vi "20150818 Main structure.vi"() -> ()   [LabVIEW 2013]
uses:
  <vilib>/Utility/error.llb/Error Cluster From Error Code.vi
  <vilib>/ErrorRing/Error Ring.xnode
  <userlib>/support/Message Queue/Message Queue.lvlib
panel:
  out "Distance(cm)":dbl
  out "UL sensor Initialize OK?":bool
  out "Servo Initialize OK?":bool
  in  "Initialize":bool
  in  "stop":bool
  out "error out":errorcluster
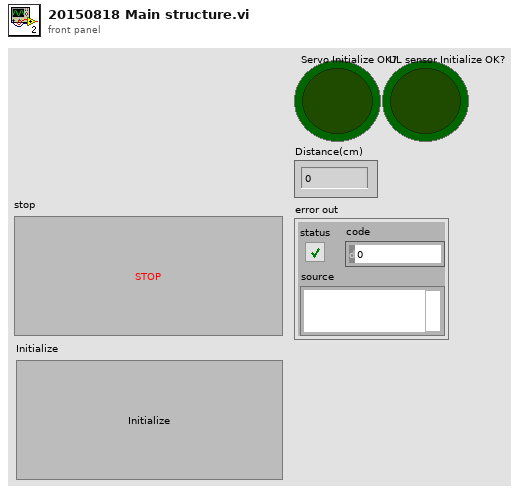
[diagram p1: front panel]
types:
  T1 = typedef "Message Queue.lvlib/All Message Queues.ctl" = cluster{"Actuator":refnum<queue>, "Sensor":refnum<queue>, "Algorithm":refnum<queue>}
  T2 = enum16{"Initialize", "Close", "Set Pulse widths"}
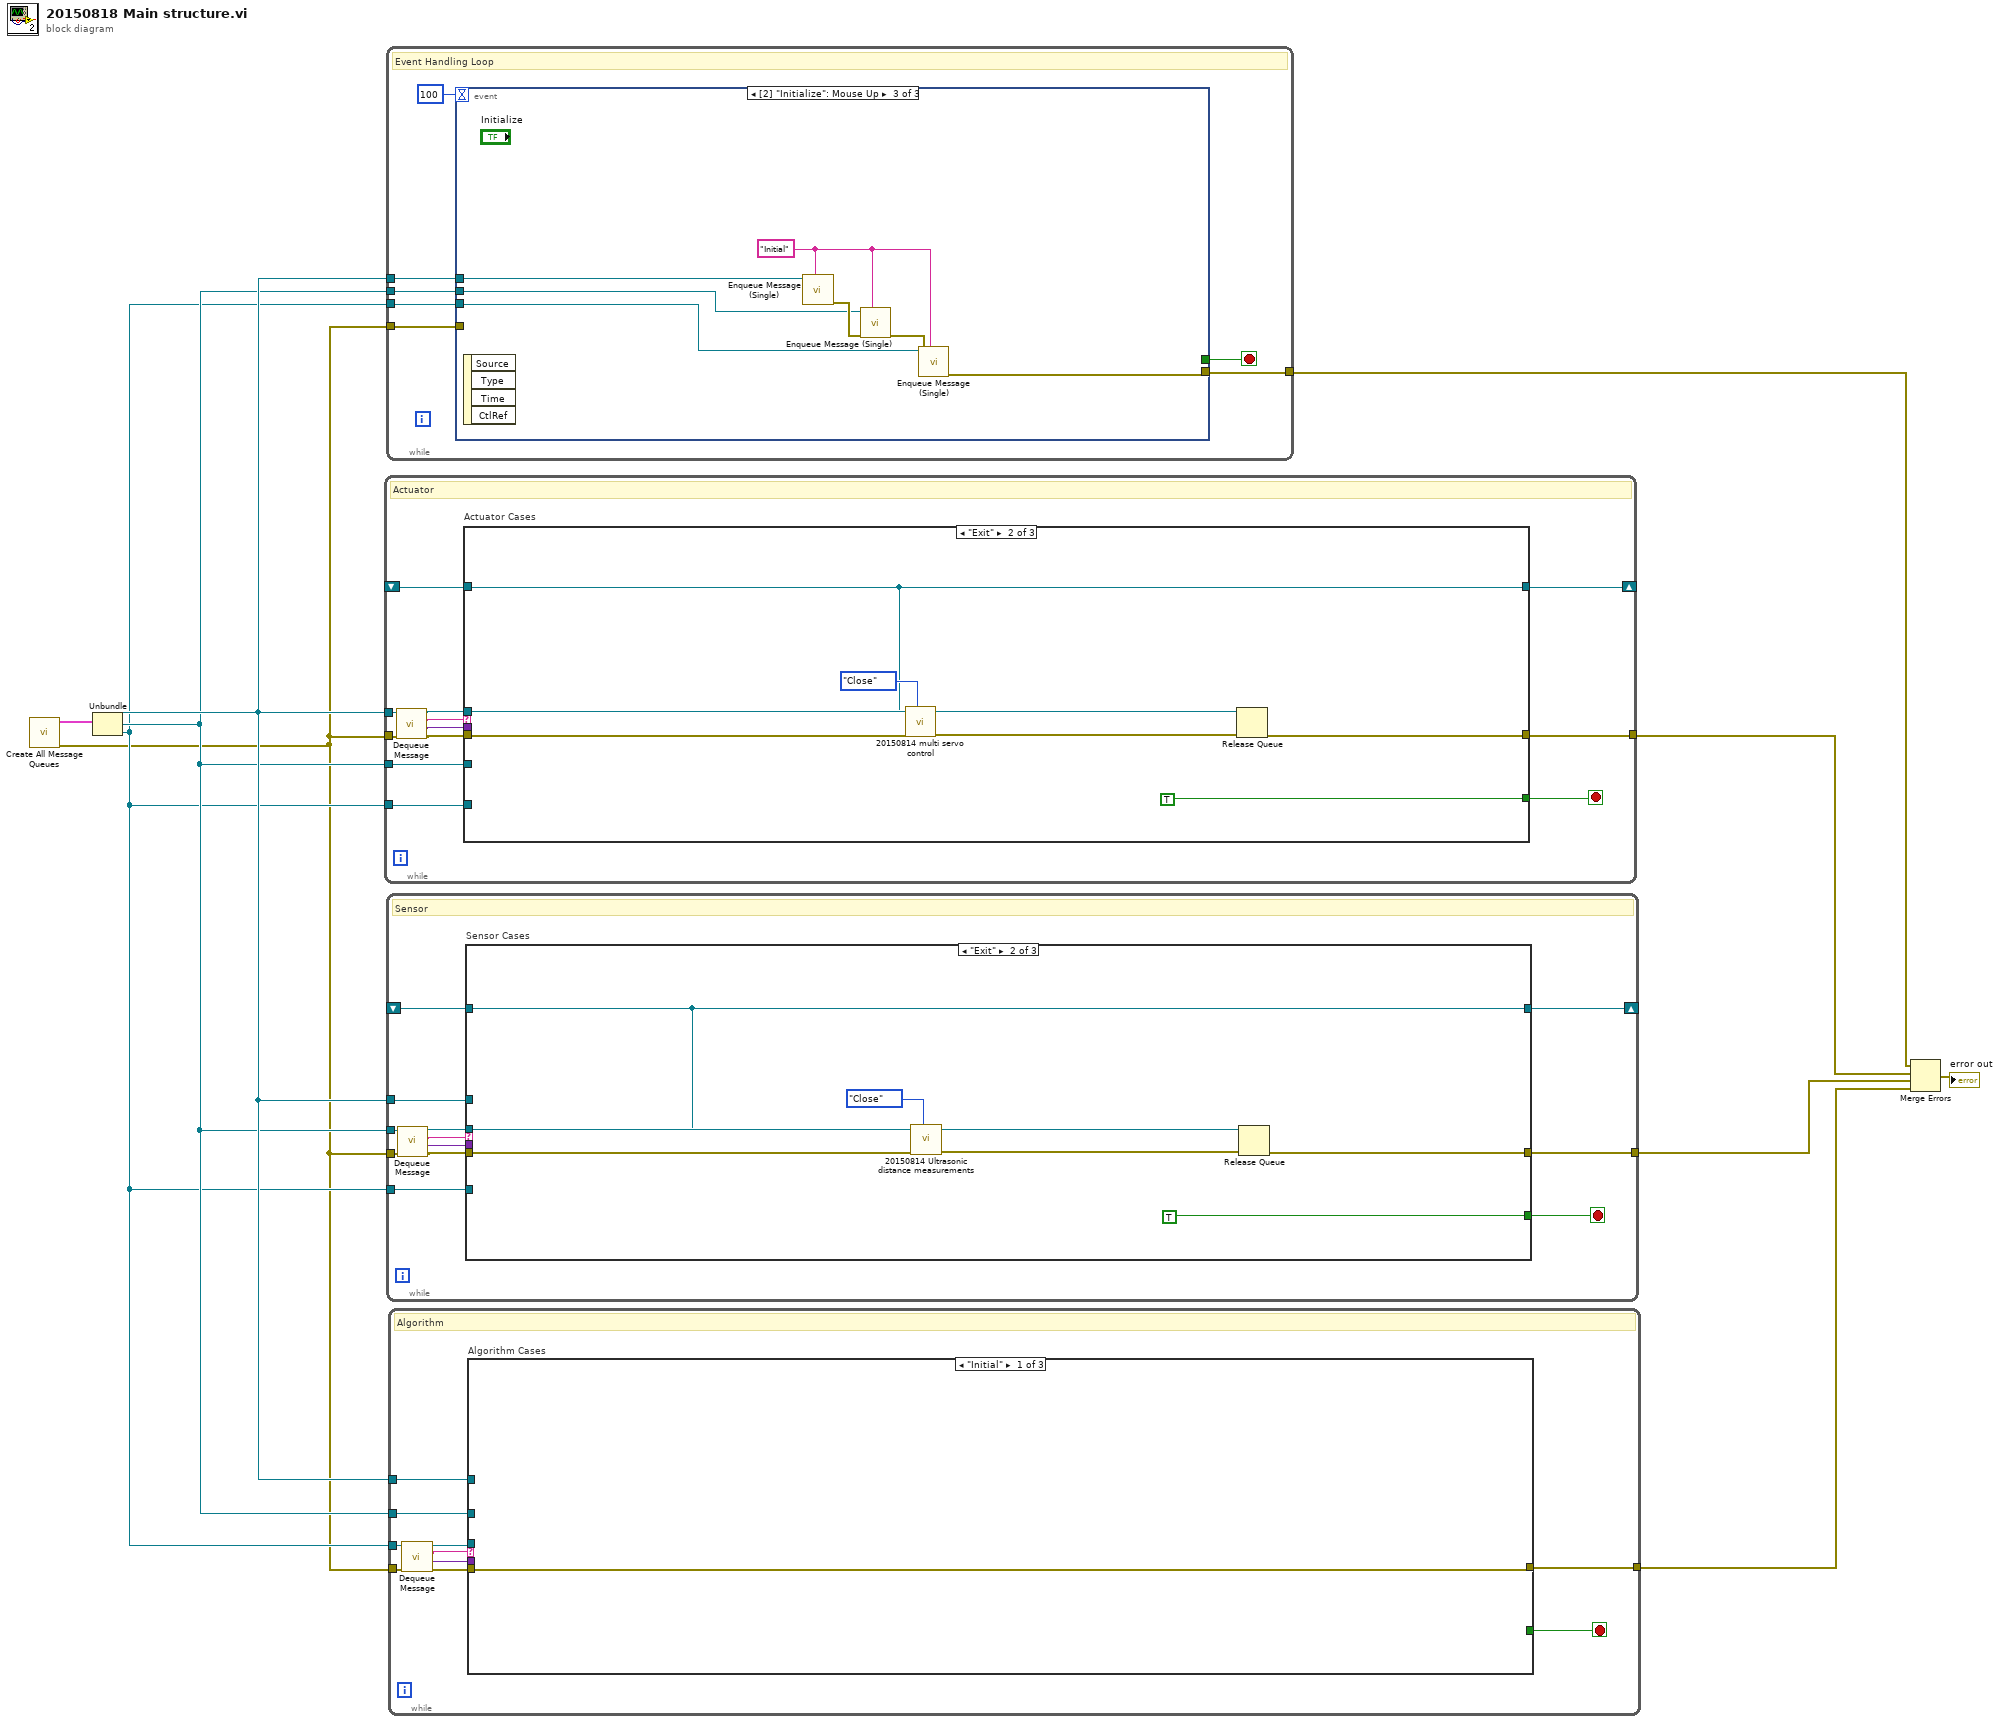
[diagram p0: block diagram]
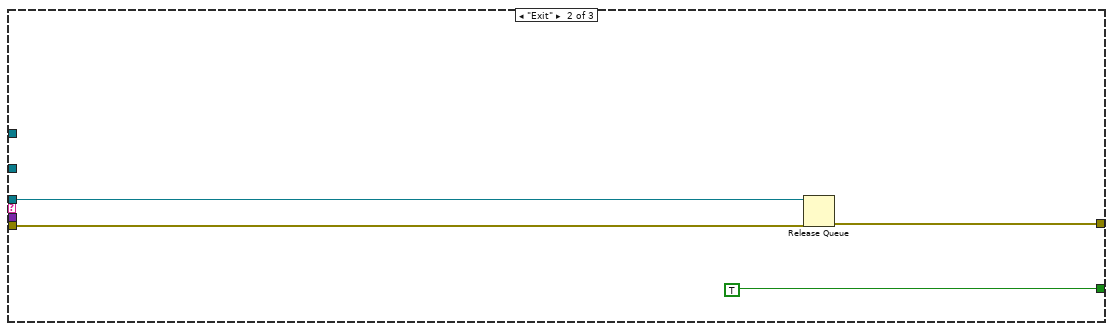
[diagram p2: hidden frame]
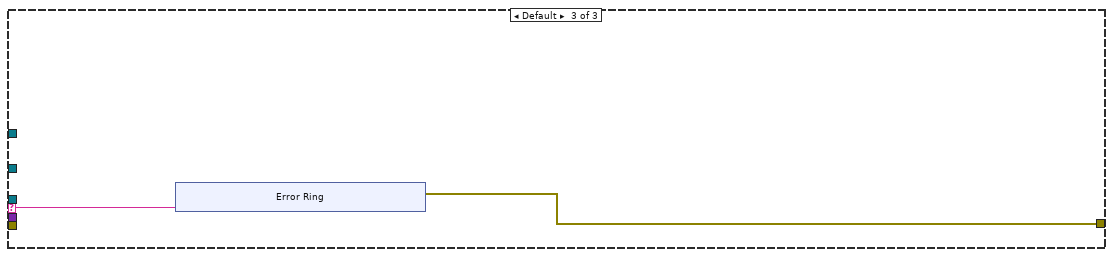
[diagram p3: hidden frame]
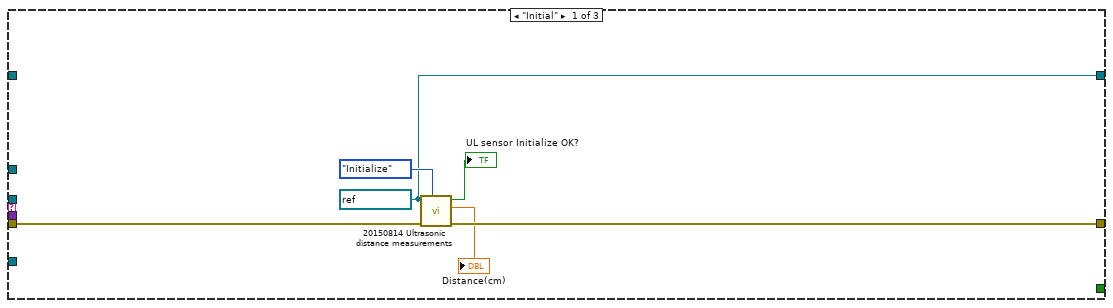
[diagram p4: hidden frame]
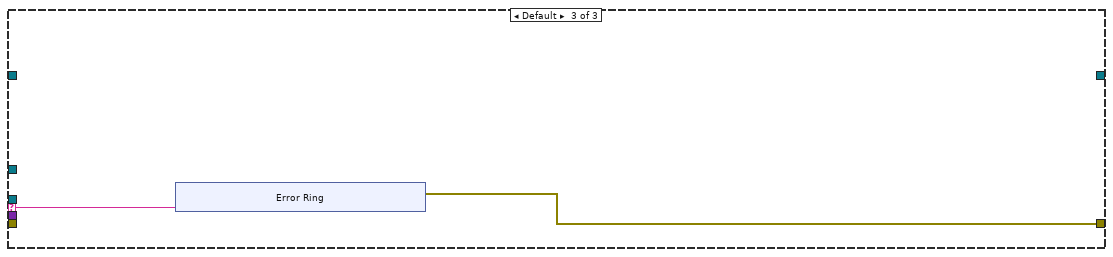
[diagram p5: hidden frame]
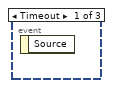
[diagram p6: hidden frame]
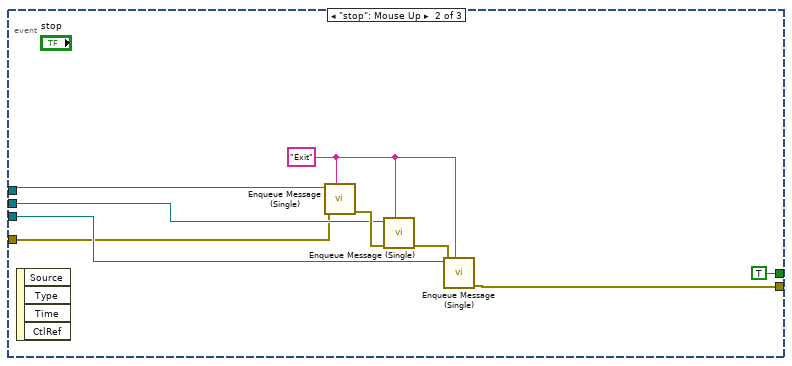
[diagram p7: hidden frame]
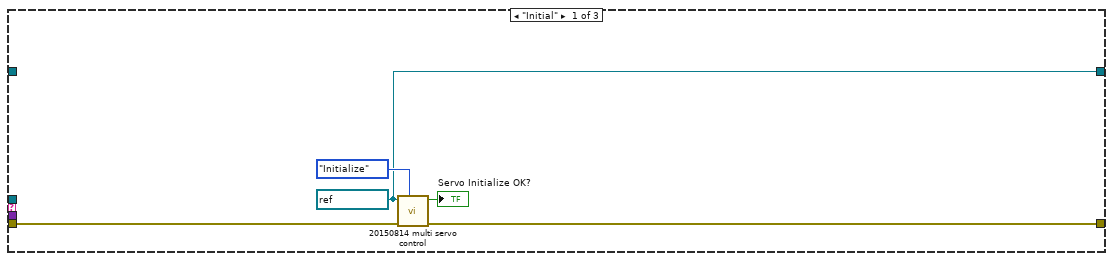
[diagram p8: hidden frame]
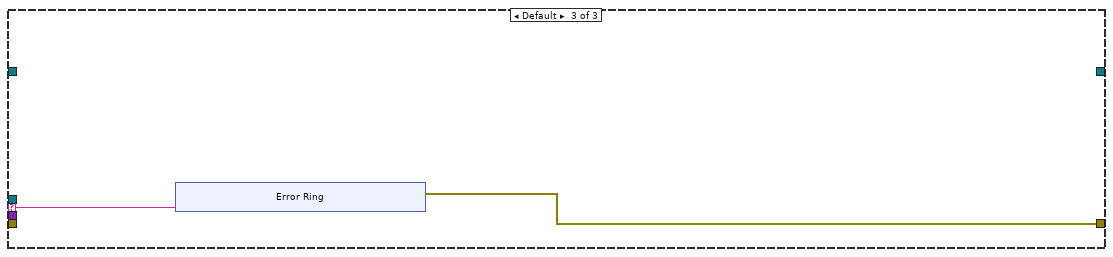
[diagram p9: hidden frame]
diagram:
  n1 = call <userlib>:"Create All Message Queues.vi"() -> ("error out"=w2:errorcluster, "Message Queues out"=w10:T1)  [unwired: 10 in]
  n2 = Unbundle(w10) -> ("Actuator"=w5:refnum<queue>, "Sensor"=w4:refnum<queue>, "Algorithm"=w3:refnum<queue>)
  n3 = while {
    tunnel: [w16] -> w9
    tunnel: w5 -> [w21]
    tunnel: w2 -> [w15]
    tunnel: w4 -> [w14]
    tunnel: w3 -> [w13]
    shift-right: [w12] -> _
    shift-left: _ -> [w11]
    stop <- w22 stop-if-true
    # "Actuator"
    n4 = call <userlib>:"Dequeue Message.vi"("error in (no error)"=w15, "Message Queue"=w21) -> ("error out"=w18:errorcluster, "Message Data"=w19:variant, "Message"=w20:string, "dup Message Queue"=w17:refnum<queue>)  [unwired: 6 in]
    n5 = case "Actuator Cases" shown="\"Exit\"" w20 {
      selector: w20 -> [_ _ w35]
      tunnel: w17 -> [_ w34 _]
      tunnel: w18 -> [w25 w31 _]
      tunnel: [w24 w33 w36] -> w16
      tunnel: [_ TRUE ("Priority Message? (F)") _] -> w22
      tunnel: w19 -> [_ _ _]
      tunnel: w14 -> [_ _ _]
      tunnel: w13 -> [_ _ _]
      tunnel: [w23 w28 _] -> w12
      tunnel: w11 -> [_ w28 _]
      frame "Initial" {
        w23 = refnum<visa-resource-name> "COM10" ("Serial Port")
        # "Initialize - Send separate messages to initialize the data and the front panel.  Bundle control references."
        n6 = call "20150814 multi servo control.vi"("Action"=T2."Initialize", "error in (no error)"=w25, "Serial Port"=w23) -> ("Error Out"=w24:errorcluster, "Initialize OK?"=→"Servo Initialize OK?":bool)  [unwired: 7 in]
      }
      frame "Exit" {
        # "Exit - Exit the application."
        n7 = call "20150814 multi servo control.vi"("Action"=T2."Close", "error in (no error)"=w31, "Serial Port"=w28) -> ("Error Out"=w30:errorcluster)  [unwired: 7 in, 1 out]
        n8 = Release Queue(queue=w34, error in (no error)=w30) -> (error out=w33:errorcluster)  [unwired: 1 in, 2 out]
      }
      frame Default {
        # "'Default' case only runs if there is a message that isn't defined in any of the other cases.  Output a programming error."
        n9 = xnode "Error Ring"("parameter 0"=w35) -> ("error out"=w36:errorcluster)
      }
    }
  }
  n10 = while {
    tunnel: w5 -> [w50]
    tunnel: w4 -> [w46]
    tunnel: w3 -> [w48]
    tunnel: w2 -> [w45]
    tunnel: [w44] -> w1
    stop <- w49 stop-if-true
    # "Event Handling Loop"
    n11 = event shown="[2] \"Initialize\": Mouse Up" {
      selector: _ -> [_ _ _]
      dyn-events: _ -> [_ _ _]
      timeout: 100 -> [_ _ _]
      tunnel: [_ TRUE ("Priority Message? (F)") _] -> w49
      tunnel: w50 -> [_ w56 w63]
      tunnel: w46 -> [_ w55 w62]
      tunnel: w48 -> [_ w54 w61]
      tunnel: w45 -> [_ w52 _]
      tunnel: [_ w51 w60] -> w44
      event Timeout {
        n12 = event-data() -> ()  [unwired: 1 in, 1 out]
      }
      event "stop": Mouse Up {
        w53 = "Exit" ("Message")
        n13 = event-data() -> ()  [unwired: 1 in, 4 out]
        n14 = call <userlib>:"Enqueue Message (Single).vi"("Message"=w53, "error in (no error)"=w52, "Message Queue"=w56) -> ("error out"=w58:errorcluster)  [unwired: 7 in, 1 out]
        n15 = call <userlib>:"Enqueue Message (Single).vi"("Message"=w53, "error in (no error)"=w58, "Message Queue"=w55) -> ("error out"=w57:errorcluster)  [unwired: 7 in, 1 out]
        n16 = call <userlib>:"Enqueue Message (Single).vi"("Message"=w53, "error in (no error)"=w57, "Message Queue"=w54) -> ("error out"=w51:errorcluster)  [unwired: 7 in, 1 out]
      }
      event "Initialize": Mouse Up {
        w64 = "Initial" ("Message")
        n17 = event-data() -> ()  [unwired: 1 in, 4 out]
        n18 = call <userlib>:"Enqueue Message (Single).vi"("Message"=w64, "Message Queue"=w63) -> ("error out"=w66:errorcluster)  [unwired: 8 in, 1 out]
        n19 = call <userlib>:"Enqueue Message (Single).vi"("Message"=w64, "error in (no error)"=w66, "Message Queue"=w62) -> ("error out"=w65:errorcluster)  [unwired: 7 in, 1 out]
        n20 = call <userlib>:"Enqueue Message (Single).vi"("Message"=w64, "error in (no error)"=w65, "Message Queue"=w61) -> ("error out"=w60:errorcluster)  [unwired: 7 in, 1 out]
      }
    }
  }
  n21 = while {
    tunnel: [w72] -> w8
    tunnel: w4 -> [w77]
    tunnel: w2 -> [w71]
    tunnel: w5 -> [w70]
    tunnel: w3 -> [w69]
    shift-right: [w68] -> _
    shift-left: _ -> [w67]
    stop <- w78 stop-if-true
    # "Sensor"
    n22 = call <userlib>:"Dequeue Message.vi"("error in (no error)"=w71, "Message Queue"=w77) -> ("error out"=w74:errorcluster, "Message Data"=w75:variant, "Message"=w76:string, "dup Message Queue"=w73:refnum<queue>)  [unwired: 6 in]
    n23 = case "Sensor Cases" shown="\"Exit\"" w76 {
      selector: w76 -> [_ _ w92]
      tunnel: w73 -> [_ w91 _]
      tunnel: w74 -> [w84 w88 _]
      tunnel: [w83 w90 w93] -> w72
      tunnel: [_ TRUE ("Priority Message? (F)") _] -> w78
      tunnel: w75 -> [_ _ _]
      tunnel: w70 -> [_ _ _]
      tunnel: w69 -> [_ _ _]
      tunnel: [w79 w85 _] -> w68
      tunnel: w67 -> [_ w85 _]
      frame "Initial" {
        w79 = refnum<visa-resource-name> "COM10" ("Serial Port")
        # "Initialize - Send separate messages to initialize the data and the front panel.  Bundle control references."
        n24 = call "20150814 Ultrasonic distance measurements.vi"("Action"=enum16{"Initialize", "Close", "Read distance"}."Initialize", "error in (no error)"=w84, "Serial Port"=w79) -> ("Error Out"=w83:errorcluster, "Distance(cm)"=→"Distance(cm)":dbl, "Initialize OK?"=→"UL sensor Initialize OK?":bool)  [unwired: 6 in]
      }
      frame "Exit" {
        # "Exit - Exit the application."
        n25 = call "20150814 Ultrasonic distance measurements.vi"("Action"=enum16{"Initialize", "Close", "Read distance"}."Close", "error in (no error)"=w88, "Serial Port"=w85) -> ("Error Out"=w87:errorcluster)  [unwired: 6 in, 2 out]
        n26 = Release Queue(queue=w91, error in (no error)=w87) -> (error out=w90:errorcluster)  [unwired: 1 in, 2 out]
      }
      frame Default {
        # "'Default' case only runs if there is a message that isn't defined in any of the other cases.  Output a programming error."
        n27 = xnode "Error Ring"("parameter 0"=w92) -> ("error out"=w93:errorcluster)
      }
    }
  }
  n28 = while {
    tunnel: [w104] -> w7
    tunnel: w3 -> [w109]
    tunnel: w2 -> [w103]
    tunnel: w5 -> [w102]
    tunnel: w4 -> [w101]
    stop <- w110 stop-if-true
    # "Algorithm"
    n29 = call <userlib>:"Dequeue Message.vi"("error in (no error)"=w103, "Message Queue"=w109) -> ("error out"=w106:errorcluster, "Message Data"=w105:variant, "Message"=w107:string, "dup Message Queue"=w108:refnum<queue>)  [unwired: 6 in]
    n30 = case "Algorithm Cases" shown="\"Initial\"" w107 {
      selector: w107 -> [_ _ w116]
      tunnel: w108 -> [_ w115 _]
      tunnel: w106 -> [w111 w112 _]
      tunnel: [w111 w114 w117] -> w104
      tunnel: [_ TRUE ("Priority Message? (F)") _] -> w110
      tunnel: w105 -> [_ _ _]
      tunnel: w102 -> [_ _ _]
      tunnel: w101 -> [_ _ _]
      frame "Initial" {
        # "Initialize - Send separate messages to initialize the data and the front panel.  Bundle control references."
      }
      frame "Exit" {
        # "Exit - Exit the application."
        n31 = Release Queue(queue=w115, error in (no error)=w112) -> (error out=w114:errorcluster)  [unwired: 1 in, 2 out]
      }
      frame Default {
        # "'Default' case only runs if there is a message that isn't defined in any of the other cases.  Output a programming error."
        n32 = xnode "Error Ring"("parameter 0"=w116) -> ("error out"=w117:errorcluster)
      }
    }
  }
  n33 = Merge Errors(w1, w9, w8, w7) -> (→"error out":errorcluster)
